vi "AngleSteam.vi"(8 "error in":errorcluster, 11 "appended array":dbl[][](array[numeric])) -> (0 "error out":errorcluster, 3 "Angle":dbl)   [LabVIEW 2019]
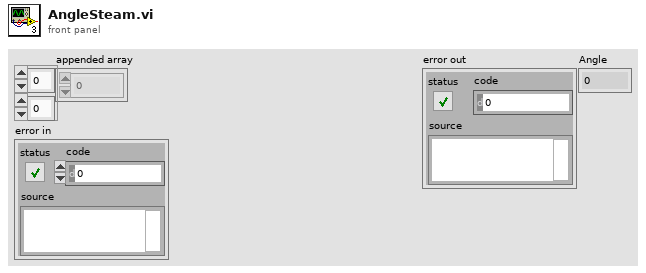
[diagram p1: front panel]
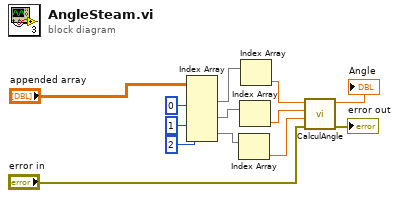
[diagram p0: block diagram]
diagram:
  n1 = Index Array(array="appended array", index (col) #1=0 ("disabled index (col)"), index (col) #2=1 ("index (col)"), index (col) #3=2 ("index (col)")) -> (element #1=w9:dbl[], element #2=w4:dbl[], element #3=w7:dbl[])  [unwired: 3 in]
  n2 = Index Array(array=w7) -> (element=w6:dbl)  [unwired: 1 in]
  n3 = Index Array(array=w4) -> (element=w5:dbl)  [unwired: 1 in]
  n4 = Index Array(array=w9) -> (element=w8:dbl)  [unwired: 1 in]
  n5 = call "CalculAngle.vi"("error constant"="error in", "Zaxis"=w6, "Yaxis"=w5, "Xaxis"=w8) -> ("error constant 2"=→"error out":errorcluster, "Numeric"=→"Angle":dbl)  [unwired: 6 in]
